vi "GetSpectrum.vi"(8 "error in (no error)":errorcluster, 11 "KeysightN9020B in":refnum<class "KeysightN9020B.lvclass">) -> (0 "error out":errorcluster, 3 "KeysightN9020B out":refnum<class "KeysightN9020B.lvclass">)   [LabVIEW 2023, in "KeysightN9020B.lvlib" / "KeysightN9020B.lvclass"]
uses:
  KeysightN9020B.lvclass
  KeysightN9020B.lvclass/KeysightN9020B.ctl
  Interfaces/AbstractInstrumentClasses/SpectrumAnalyzer_LV/SpectrumAnalyzerComm/SpectrumAnalyzerComm Messages/SpectrumAcquired Msg/SpectrumAcquired Msg.lvclass
  <vilib>/ActorFramework/Actor/Actor.lvclass
  C:/Program Files/National Instruments/LabVIEW 2023/vi.lib/ActorFramework/Actor/Actor.lvclass
  C:/Users/Administrator/Documents/LVDAQ/ConcreteClasses/ConcreteInstrumentClasses/KeysightN9020B/KeysightN9020B.lvclass
  C:/Users/Administrator/Documents/LVDAQ/Interfaces/InitDeinitInterface/InitDeinit/InitDeinit.lvclass
  C:/Users/Administrator/Documents/LVDAQ/Interfaces/AbstractInstrumentClasses/SpectrumAnalyzer_LV/SpectrumAnalyzerInterface/SpectrumAnalyzer.lvclass
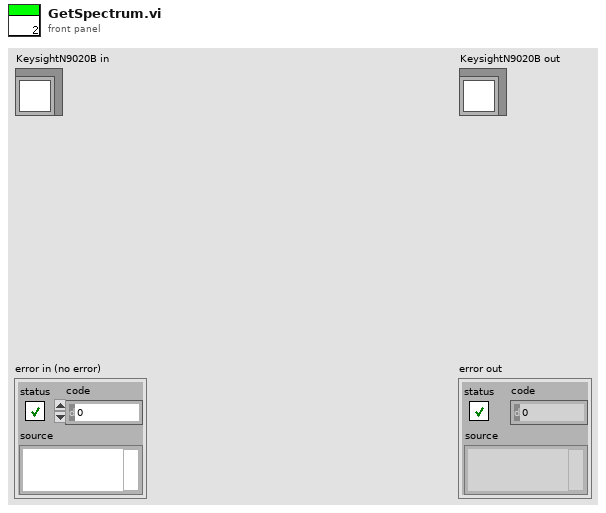
[diagram p1: front panel]
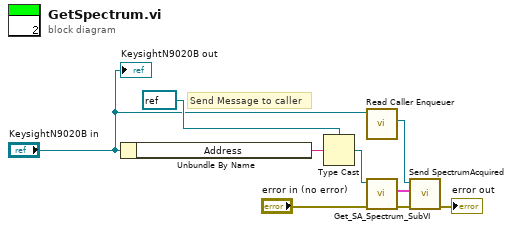
[diagram p0: block diagram]
diagram:
  # "Send Message to caller"
  n1 = Unbundle By Name("KeysightN9020B in") -> ("Address"=w8:string)
  n2 = Type Cast(type=refnum<k15> refnum ("IVI Refnum in"), x=w8) -> (*(type *) &x=w6:refnum<k15>)
  n3 = call <vilib>:"Read Caller Enqueuer.vi"("Actor"="KeysightN9020B in") -> ("Caller Enqueuer"=w3:refnum<class "Message Enqueuer.lvclass">)  [unwired: 10 in]
  n4 = call "Get_SA_Spectrum_SubVI.vi"("error in (no error)"="error in (no error)", "IVI Refnum in"=w6) -> ("error out"=w2:errorcluster, "Spectrum"=w5:cluster{"Frequency":dbl[], "Amplitude":dbl[]})  [unwired: 7 in, 1 out]
  n5 = call "Send SpectrumAcquired.vi"("error in (no error)"=w2, "Spectrum"=w5, "Message Enqueuer"=w3) -> ("error out"=→"error out":errorcluster)  [unwired: 7 in, 1 out]
  "KeysightN9020B out" <- "KeysightN9020B in"
